vi "Revisar Fechas.vi"(8 "error in (no error)":errorcluster, 10 "End Time":timestamp, 11 "Start Time":timestamp) -> (0 "error out":errorcluster, 1 "Suma":dbl, 2 "Column Names":string[](array[string]), 3 "Result Set":string[][](table) caption="Table Servicios")   [LabVIEW 2020, in "UI.lvlib"]
uses:
  <vilib>/drjdpowell/SQLite Library/SQL Connection/Open (path).vi
  <vilib>/drjdpowell/SQLite Library/SQL Connection/Open (string).vi
  <vilib>/AdvancedString/Path To Command Line String.vi
  <vilib>/drjdpowell/SQLite Library/SQL Connection/Execute SQL.vi
  <vilib>/drjdpowell/SQLite Library/SQL Connection/Connection.lvclass
  UI.lvlib
  <vilib>/drjdpowell/SQLite Library/SQLite.lvlib
  Contabilidad/Contabilidad.lvlib
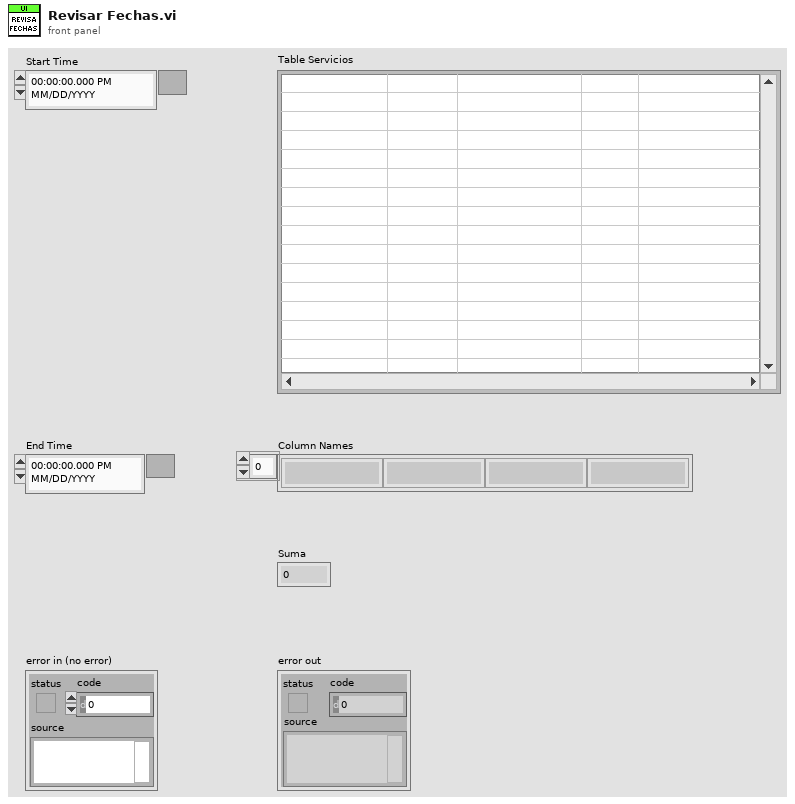
[diagram p1: front panel]
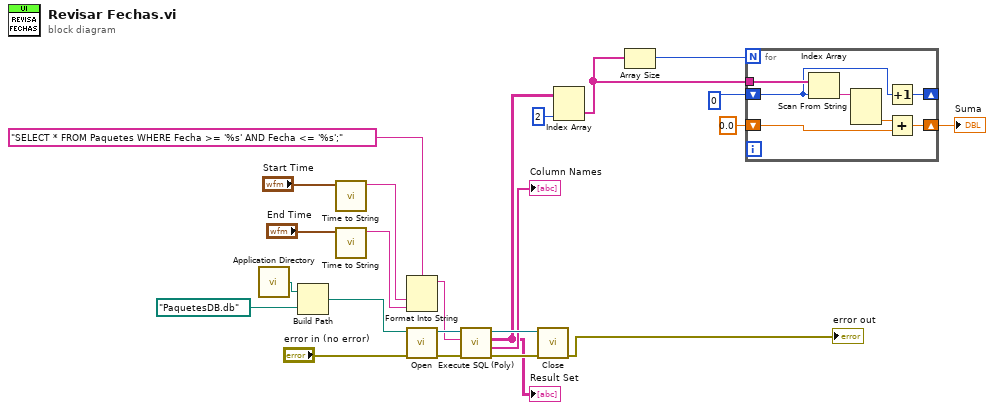
[diagram p0: block diagram]
diagram:
  n1 = call <vilib>:"Application Directory.vi"() -> ("Application Directory"=w16:path)
  n2 = Build Path(base path=w16, name or relative path=path "PaquetesDB.db") -> (appended path=w14:path)
  n3 = call "Time to String.vi"("Time"="Start Time") -> ("date/time string"=w11:string)  [unwired: 10 in]
  n4 = call "Time to String.vi"("Time"="End Time") -> ("date/time string"=w9:string)  [unwired: 10 in]
  n5 = Format Into String(format string="SELECT * FROM Paquetes WHERE Fecha >= '%s' AND Fecha <= '%s';", w11, w9) -> (resulting string=w17:string)  [unwired: 2 in, 1 out]
  n6 = call-poly <vilib>:"Open.vi"("error in (no error)"="error in (no error)", "db file"=w14) -> ("error out"=w23:errorcluster, "SQLite Connection"=w20:refnum<class "Connection.lvclass">)  [unwired: 8 in]
  n7 = call-poly <vilib>:"Execute SQL (Poly).vi"("error in (no error)"=w23, "SQL"=w17, "SQLite Connection in"=w20) -> ("error out"=w21:errorcluster, "Column Names"=→"Column Names":string[], "Result Set"=w8:string[][], "SQLite Connection"=w22:refnum<class "Connection.lvclass">)  [unwired: 5 in]
  "Result Set" <- w8
  n8 = call-dynamic "Close.vi"("error in (no error)"=w21, "SQLite Connection in"=w22) -> ("error out"=→"error out":errorcluster)  [unwired: 9 in]
  n9 = Index Array(array=w8, index (col)=2 ("disabled index (col)")) -> (element=w6:string[])  [unwired: 1 in]
  n10 = Array Size(array=w6) -> (size(s)=w5:i32)
  n11 = for {
    N: w5 -> [_]
    tunnel: w6 -> [w30]
    shift-right: [w29] -> _
    shift-left: 0 -> [w28]
    shift-right: [w24] -> w3
    shift-left: 0.0 -> [w25]
    n12 = Index Array(array=w30, index=w28) -> (element=w27:string)
    n13 = Scan From String(input string=w27) -> (output 1=w26:dbl)  [unwired: 4 in, 3 out]
    n14 = Increment(x=w28) -> (x+1=w29:i32)
    n15 = Add(x=w26, y=w25) -> (x+y=w24:dbl)
  }
  "Suma" <- w3
